vi "pco.camera_Avg_Example_IMAQ.vi"() -> ()   [LabVIEW 2019]
uses:
  pco.camera/Camera.lvclass
panel:
  out "rawImage":u16[][](array[numeric])
  out "Image":T1(plugin-control)
  in  "data_format":T2(ring)=enum."Mono16"
  out "Recorded Images":u32
  in  "Quit":bool
  in  "roiY1":u64=2 min=2 max=1040 step=1
  in  "roiX1":u64=2 min=2 max=1392 step=1
  in  "roiY0":u64=1 min=1 max=1039 step=1
  in  "roiX0":u64=1 min=1 max=1391 step=1
  out "Image Height":u64
  out "Image Width":u64
  in  "dwImgCount":u32=10 caption="Required Number of Images" max=4023
  out "Error":errorcluster {"code" format="%x"}
  # "This example shows how to continously compute and show an averaged image.\nHere the camera class is operated in sequence mode and the required number of images also defines the number of images that will be averaged\nIt is a good starting point for writing own applications.\nBut it will not be fail save, i.e. doesnt react on errors, just handles them forward to the end\n\nUsage:\nSelect your required image count you want to average over before you start the program.\nOnce started, the camera class will be initialized and image record will start automatically.\nInside the acquisition loop the program will record the image sequence.\nThen it calculates the average image and shows it.\nBy using the ROI parameters you can crop the image to select certain regions\n\nBy clicking Quit Application the record will stop and will force an exit of the camera class"
  # "pco.labview"
  # "Camera Setup"
  # "Recording Control"
  # "Parameters for image readout"
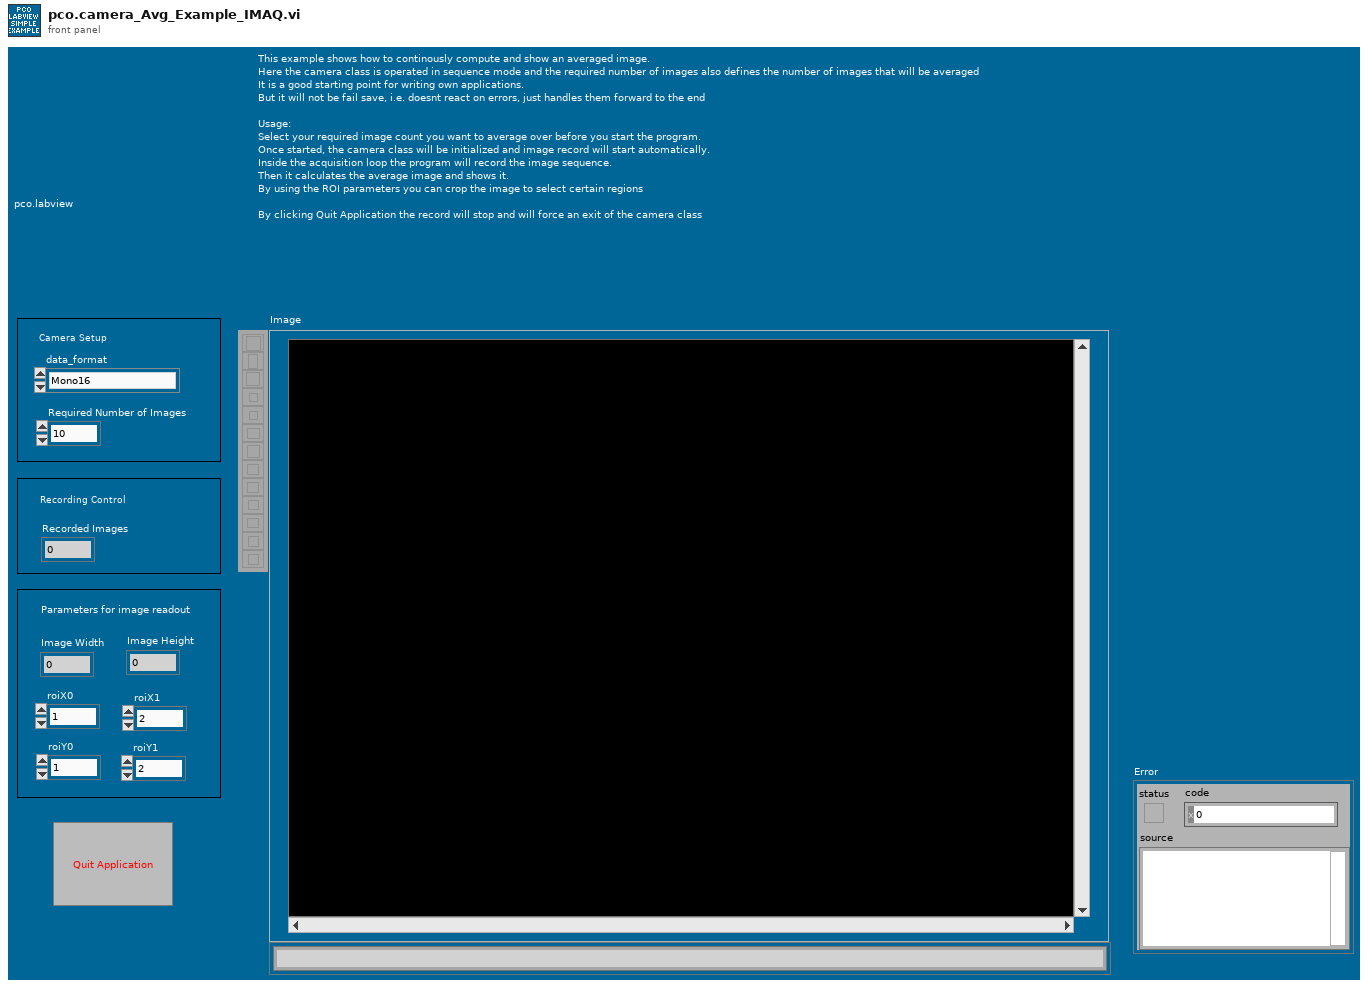
[diagram p1: front panel]
types:
  T1 = typedef "IMAQ Image.ctl" = refnum<image>
  T2 = enum16{"Undefined", "Mono8", "Mono16", "BGRA8", "RGBA8", "BGRA16", "RGBA16", "CompressedMono8"}
  T3 = enum8{"Enabled", "Disabled", "Disabled and Grayed Out"}
  T4 = enum16{"sequence", "sequence non blocking", "ring buffer", "fifo", "sequence_dpcore", "sequence_non_blocking_dpcore", "ring_buffer_dpcore", "fifo_dpcore", "tif", "multitif", "pcoraw", "b16", "dicom", "multidicom"}
  T5 = typedef "Image Type" = u32
  T6 = typedef "Camera.lvclass/binning.ctl" = cluster{"vert":u16, "horz":u16}
  T7 = cluster{"exposure_time_s":dbl, "delay_time_s":dbl, "roi":cluster{"x0":u64, "y0":u64, "x1":u64, "y1":u64}, "timestamp_mode":u16, "pixelrate":u32, "trigger_mode":u16, "acquire_mode":u16, "metadata_mode":u16, "noisefilter_mode":u16, "binning":T6}
  T8 = typedef "Color (U64)" = cluster{"Plane 3 (Blue)":u16, "Plane 2 (Green)":u16, "Plane 1 (Red)":u16, "Plane 4 (alpha)":u16}
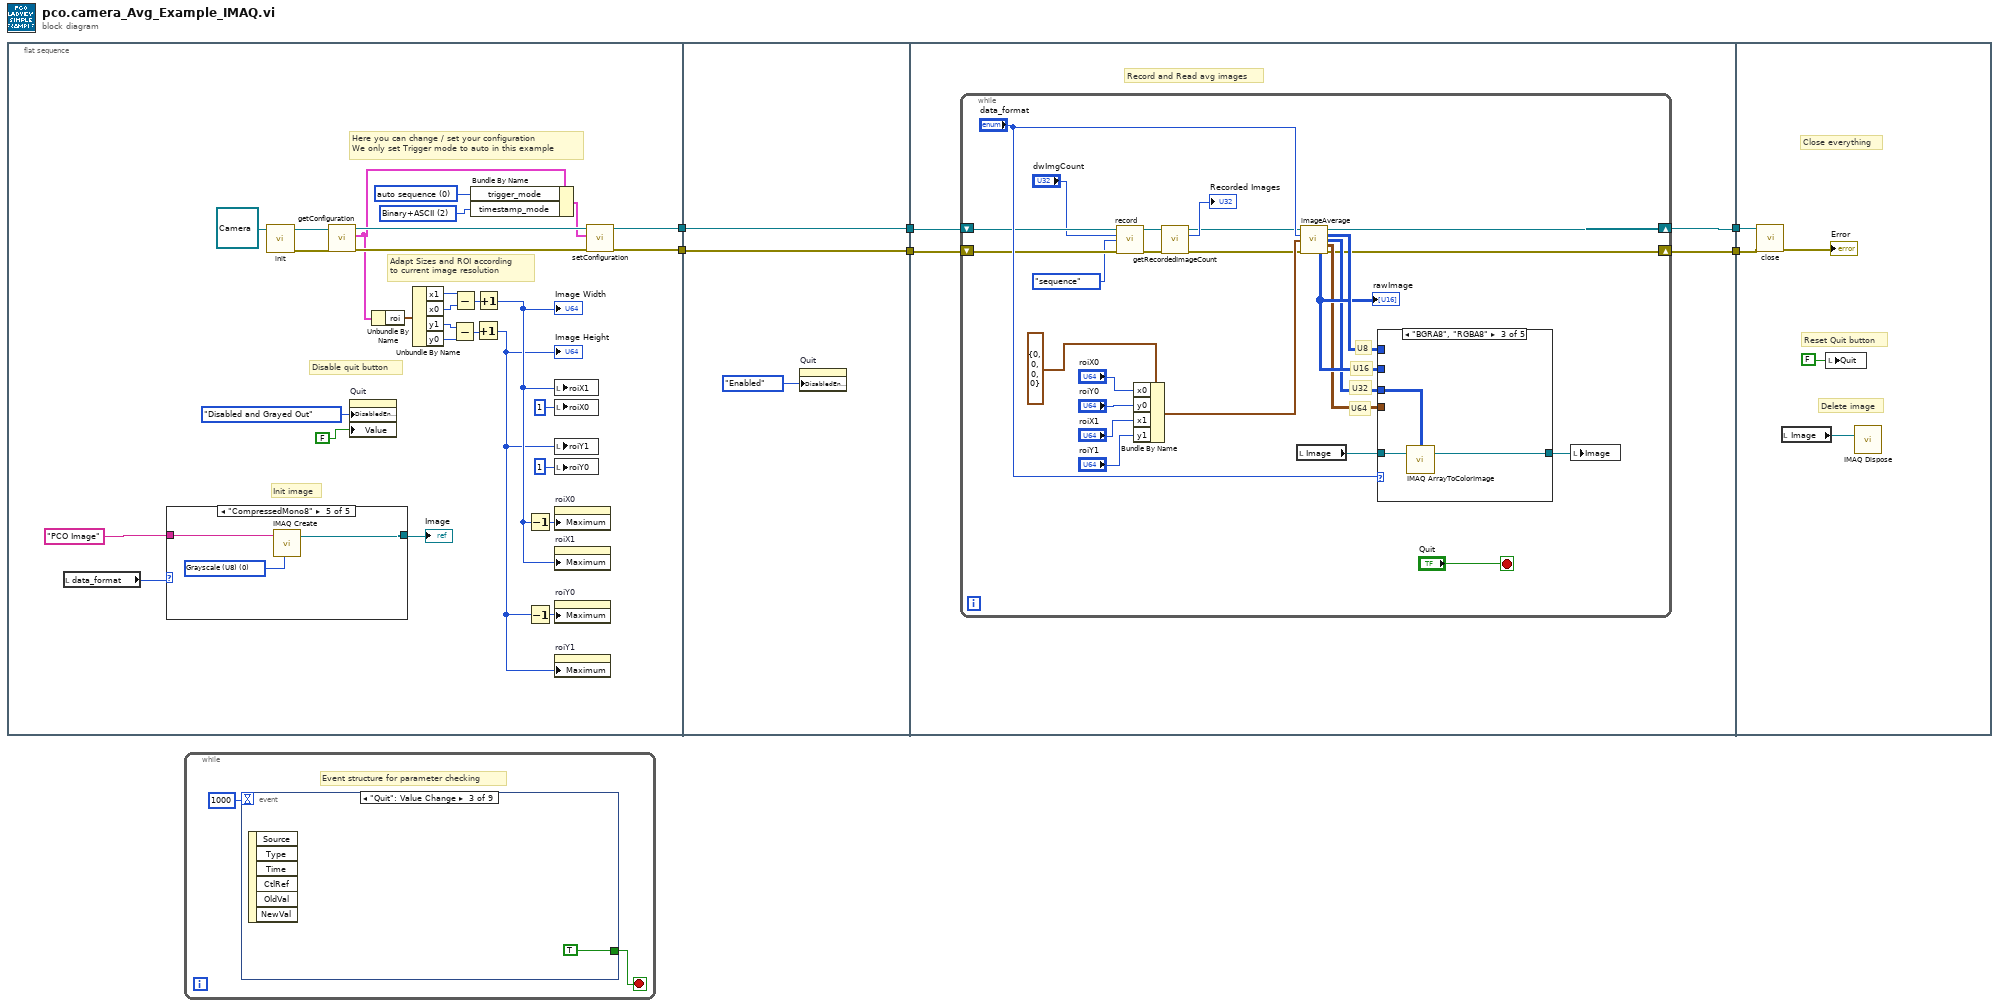
[diagram p0: block diagram]
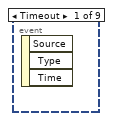
[diagram p2: hidden frame]
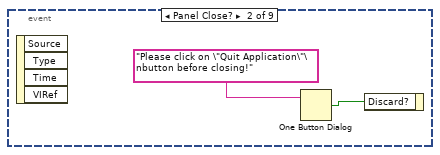
[diagram p3: hidden frame]
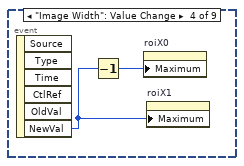
[diagram p4: hidden frame]
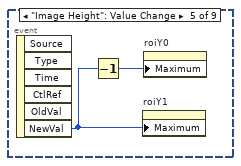
[diagram p5: hidden frame]
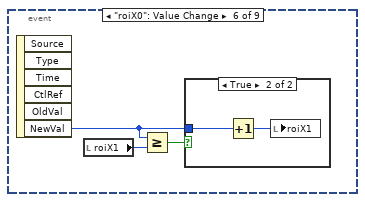
[diagram p6: hidden frame]
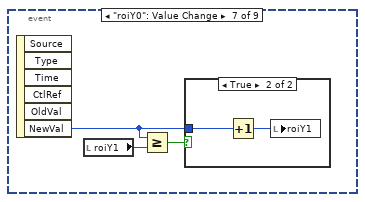
[diagram p8: hidden frame]
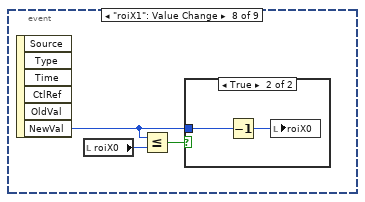
[diagram p10: hidden frame]
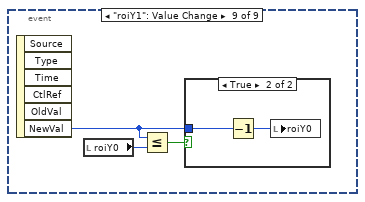
[diagram p12: hidden frame]
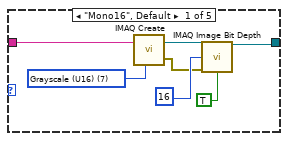
[diagram p14: hidden frame]
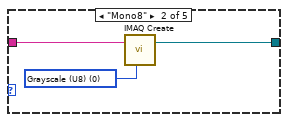
[diagram p15: hidden frame]
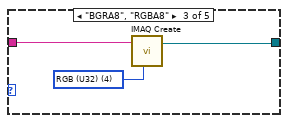
[diagram p16: hidden frame]
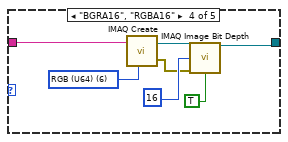
[diagram p17: hidden frame]
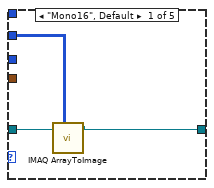
[diagram p18: hidden frame]
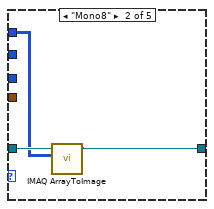
[diagram p19: hidden frame]
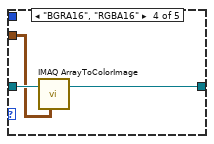
[diagram p20: hidden frame]
diagram:
  n1 = flat-sequence {
    tunnel: [w8] -> w6
    tunnel: [w7] -> w5
    tunnel: w6 -> [w60]
    tunnel: w5 -> [w59]
    tunnel: [w60] -> w4
    tunnel: [w59] -> w3
    tunnel: [w65] -> w2
    tunnel: [w64] -> w1
    tunnel: w3 -> [w63]
    tunnel: w4 -> [w62]
    tunnel: w2 -> [w108]
    tunnel: w1 -> [w107]
    frame #0 {
      w14 = u16 2 items=["OFF", "Binary", "Binary+ASCII", "ASCII"] ("TimestampMode")
      w32 = u16 0 items=["auto sequence"=0, "software trigger"=1, "external exposure start & software trigger"=2, "external exposure control"=3, "external synchronized"=4, "fast external exposure control"=5, "external CDS control"=6, "slow external exposure control"=7, "external synchronized HDSDI"=258] ("TriggerMode")
      # "Init image"
      # "Adapt Sizes and ROI according\nto current image resolution"
      # "Disable quit button"
      # "Here you can change / set your configuration\nWe only set Trigger mode to auto in this example"
      n2 = local read "data_format"() -> (w11:T2)
      n3 = case shown="\"CompressedMono8\"" w11 {
        tunnel: "PCO Image" ("Image Name") -> [w41 w45 w47 w54 w57]
        tunnel: [w36 w43 w46 w49 w56] -> w10
        frame "Mono16", Default {
          w42 = T5 7 items=["Grayscale (U8)", "Grayscale (I16)", "Grayscale (SGL)", "Complex (CSG)", "RGB (U32)", "HSL (U32)", "RGB (U64)", "Grayscale (U16)"] ("Image Type")
          n4 = call "IMAQ Create"("Image Name"=w41, "Image Type"=w42) -> ("New Image"=w38:T1, "error out"=w37:errorcluster)  [unwired: 3 in]
          n5 = call "IMAQ Image Bit Depth"("Image"=w38, "Bit Depth (0)"=u32 16, "error in (no error)"=w37, "Get/Set Bit Depth? (Set)"=TRUE) -> ("Image Out"=w36:T1)  [unwired: 9 in, 2 out]
        }
        frame "Mono8" {
          w44 = T5 0 items=["Grayscale (U8)", "Grayscale (I16)", "Grayscale (SGL)", "Complex (CSG)", "RGB (U32)", "HSL (U32)", "RGB (U64)", "Grayscale (U16)"] ("Image Type")
          n6 = call "IMAQ Create"("Image Name"=w45, "Image Type"=w44) -> ("New Image"=w43:T1)  [unwired: 3 in, 1 out]
        }
        frame "BGRA8", "RGBA8" {
          w48 = T5 4 items=["Grayscale (U8)", "Grayscale (I16)", "Grayscale (SGL)", "Complex (CSG)", "RGB (U32)", "HSL (U32)", "RGB (U64)", "Grayscale (U16)"] ("Image Type")
          n7 = call "IMAQ Create"("Image Name"=w47, "Image Type"=w48) -> ("New Image"=w46:T1)  [unwired: 3 in, 1 out]
        }
        frame "BGRA16", "RGBA16" {
          w55 = T5 6 items=["Grayscale (U8)", "Grayscale (I16)", "Grayscale (SGL)", "Complex (CSG)", "RGB (U32)", "HSL (U32)", "RGB (U64)", "Grayscale (U16)"] ("Image Type")
          n8 = call "IMAQ Create"("Image Name"=w54, "Image Type"=w55) -> ("New Image"=w51:T1, "error out"=w50:errorcluster)  [unwired: 3 in]
          n9 = call "IMAQ Image Bit Depth"("Image"=w51, "Bit Depth (0)"=u32 16, "error in (no error)"=w50, "Get/Set Bit Depth? (Set)"=TRUE) -> ("Image Out"=w49:T1)  [unwired: 9 in, 2 out]
        }
        frame "CompressedMono8" {
          w58 = T5 0 items=["Grayscale (U8)", "Grayscale (I16)", "Grayscale (SGL)", "Complex (CSG)", "RGB (U32)", "HSL (U32)", "RGB (U64)", "Grayscale (U16)"] ("Image Type")
          n10 = call "IMAQ Create"("Image Name"=w57, "Image Type"=w58) -> ("New Image"=w56:T1)  [unwired: 3 in, 1 out]
        }
      }
      "Image" <- w10
      n11 = call-dynamic "init.vi"("Camera in"=refnum<class "Camera.lvclass"> refnum ("PCOCamera in")) -> ("Camera out"=w34:refnum<class "Camera.lvclass">, "error out"=w33:errorcluster)  [unwired: 8 in]
      n12 = call-dynamic "getConfiguration.vi"("error in (no error)"=w33, "Camera in"=w34) -> ("error out"=w30:errorcluster, "configuration"=w24:T7, "Camera out"=w31:refnum<class "Camera.lvclass">)  [unwired: 7 in]
      n13 = property on="Quit" class="Bool (strict)"("DisabledEnum"=T3."Disabled and Grayed Out" ("Disabled"), "Value"=FALSE ("Stop")) -> ()  [unwired: 2 in, 2 out]
      n14 = Unbundle By Name(w24) -> ("roi"=w23:cluster{"x0":u64, "y0":u64, "x1":u64, "y1":u64})
      n15 = Unbundle By Name(w23) -> ("x1"=w21:u64, "x0"=w22:u64, "y1"=w19:u64, "y0"=w20:u64)
      n16 = Subtract(x=w19, y=w20) -> (x-y=w17:u64)
      n17 = Subtract(x=w21, y=w22) -> (x-y=w18:u64)
      n18 = Bundle By Name(cluster=w24, "trigger_mode"=w32, "timestamp_mode"=w14) -> (w29:T7)
      n19 = Increment(x=w17) -> (x+1=w15:u64)
      "Image Height" <- w15
      n20 = Increment(x=w18) -> (x+1=w16:u64)
      "Image Width" <- w16
      n21 = Decrement(x=w16) -> (x-1=w26:u64)
      n22 = Decrement(x=w15) -> (x-1=w25:u64)
      n23 = local write "roiX1"(w16) -> ()
      n24 = local write "roiX0"(u64 1 ("roiY0")) -> ()
      n25 = local write "roiY1"(w15) -> ()
      n26 = local write "roiY0"(u64 1 ("roiY0")) -> ()
      n27 = property on="roiX0" class="DigNum (strict)"("Maximum"=w26) -> ()  [unwired: 2 in, 2 out]
      n28 = property on="roiX1" class="DigNum (strict)"("Maximum"=w16) -> ()  [unwired: 2 in, 2 out]
      n29 = property on="roiY0" class="DigNum (strict)"("Maximum"=w25) -> ()  [unwired: 2 in, 2 out]
      n30 = property on="roiY1" class="DigNum (strict)"("Maximum"=w15) -> ()  [unwired: 2 in, 2 out]
      n31 = call-dynamic "setConfiguration.vi"("error in (no error)"=w30, "configuration"=w29, "Camera in"=w31) -> ("error out"=w7:errorcluster, "Camera out"=w8:refnum<class "Camera.lvclass">)  [unwired: 7 in]
    }
    frame #1 {
      n32 = property on="Quit" class="Bool (strict)"("DisabledEnum"=T3."Enabled" ("Disabled")) -> ()  [unwired: 2 in, 2 out]
    }
    frame #2 {
      # "Record and Read avg images"
      n33 = while {
        shift-right: [w76] -> w65
        shift-left: w62 -> [w75]
        shift-right: [w66] -> w64
        shift-left: w63 -> [w74]
        stop <- "Quit" stop-if-true
        # "U64"
        # "U32"
        # "U16"
        # "U8"
        n34 = call-dynamic "record.vi"("Camera in"=w75, "num_images"="dwImgCount", "record_mode"=T4."sequence", "error in (no error)"=w74) -> ("Camera out"=w72:refnum<class "Camera.lvclass">, "error out"=w71:errorcluster)  [unwired: 10 in]
        n35 = Bundle By Name(cluster=cluster{"x0":u64, "y0":u64, "x1":u64, "y1":u64} {"x0"=0, "y0"=0, "x1"=0, "y1"=0} ("roi"), "x0"="roiX0", "y0"="roiY0", "x1"="roiX1", "y1"="roiY1") -> (w86:cluster{"x0":u64, "y0":u64, "x1":u64, "y1":u64})
        n36 = call-dynamic "getRecordedImageCount.vi"("Camera in"=w72, "error in (no error)"=w71) -> ("Camera out"=w69:refnum<class "Camera.lvclass">, "recorded_image_count"=→"Recorded Images":u32, "error out"=w68:errorcluster)  [unwired: 11 in]
        n37 = local read "Image"() -> (w80:T1)
        n38 = call-dynamic "imageAverage.vi"("Camera in"=w69, "data_format"="data_format", "roi"=w86, "error in (no error)"=w68) -> ("Camera out"=w76:refnum<class "Camera.lvclass">, "image (U8)"=w84:u8[][], "image (U32)"=w82:u32[][], "image (U64)"=w81:T8[][], "raw_image (U16)"=w83:u16[][], "error out"=w66:errorcluster)  [unwired: 6 in]
        "rawImage" <- w83
        n39 = case shown="\"BGRA8\", \"RGBA8\"" "data_format" {
          tunnel: w80 -> [w93 w96 w99 w102 w105]
          tunnel: [w91 w94 w98 w100 w104] -> w79
          tunnel: w81 -> [_ _ _ w101 _]
          tunnel: w82 -> [_ _ w97 _ _]
          tunnel: w84 -> [_ w95 _ _ w103]
          tunnel: w83 -> [w92 _ _ _ _]
          frame "Mono16", Default {
            n40 = call "IMAQ ArrayToImage"("Image Pixels (U16)"=w92, "Image"=w93) -> ("Image Out"=w91:T1)  [unwired: 8 in, 1 out]
          }
          frame "Mono8" {
            n41 = call "IMAQ ArrayToImage"("Image Pixels (U8)"=w95, "Image"=w96) -> ("Image Out"=w94:T1)  [unwired: 8 in, 1 out]
          }
          frame "BGRA8", "RGBA8" {
            n42 = call "IMAQ ArrayToColorImage"("Image Pixels (U32)"=w97, "Image"=w99) -> ("Image Out"=w98:T1)  [unwired: 3 in, 1 out]
          }
          frame "BGRA16", "RGBA16" {
            n43 = call "IMAQ ArrayToColorImage"("Image"=w102, "Image Pixels (U64)"=w101) -> ("Image Out"=w100:T1)  [unwired: 3 in, 1 out]
          }
          frame "CompressedMono8" {
            n44 = call "IMAQ ArrayToImage"("Image Pixels (U8)"=w103, "Image"=w105) -> ("Image Out"=w104:T1)  [unwired: 8 in, 1 out]
          }
        }
        n45 = local write "Image"(w79) -> ()
      }
    }
    frame #3 {
      # "Delete image"
      # "Reset Quit button"
      # "Close everything"
      n46 = call-dynamic "close.vi"("error in (no error)"=w107, "Camera in"=w108) -> ("error out"=→"Error":errorcluster)  [unwired: 9 in]
      n47 = local read "Image"() -> (w106:T1)
      n48 = local write "Quit"(FALSE ("Stop")) -> ()
      n49 = call "IMAQ Dispose"("Image"=w106) -> ()  [unwired: 5 in, 1 out]
    }
  }
  n50 = while {
    stop <- w111 stop-if-true
    # "Event structure for parameter checking"
    n51 = event shown="[2] \"Quit\": Value Change" {
      selector: _ -> [_ _ _ _ _ _ _ _ _]
      dyn-events: _ -> [_ _ _ _ _ _ _ _ _]
      timeout: 1000 -> [_ _ _ _ _ _ _ _ _]
      tunnel: [_ _ TRUE _ _ _ _ _ _] -> w111
      event Timeout {
        n52 = event-data() -> ()  [unwired: 1 in, 3 out]
      }
      event Panel Close? {
        n53 = event-data() -> ()  [unwired: 1 in, 4 out]
        n54 = One Button Dialog(message="Please click on \"Quit Application\"\nbutton before closing!") -> (true=w113:bool)  [unwired: 1 in]
        n55 = event-data("Discard?"=w113) -> ()  [unwired: 1 in, 1 out]
      }
      event "Quit": Value Change {
        n56 = event-data() -> ()  [unwired: 1 in, 6 out]
      }
      event "Image Width": Value Change {
        n57 = event-data() -> ("NewVal"=w116:u64)  [unwired: 1 in, 5 out]
        n58 = Decrement(x=w116) -> (x-1=w117:u64)
        n59 = property on="roiX0" class="DigNum (strict)"("Maximum"=w117) -> ()  [unwired: 2 in, 2 out]
        n60 = property on="roiX1" class="DigNum (strict)"("Maximum"=w116) -> ()  [unwired: 2 in, 2 out]
      }
      event "Image Height": Value Change {
        n61 = event-data() -> ("NewVal"=w118:u64)  [unwired: 1 in, 5 out]
        n62 = Decrement(x=w118) -> (x-1=w119:u64)
        n63 = property on="roiY1" class="DigNum (strict)"("Maximum"=w118) -> ()  [unwired: 2 in, 2 out]
        n64 = property on="roiY0" class="DigNum (strict)"("Maximum"=w119) -> ()  [unwired: 2 in, 2 out]
      }
      event "roiX0": Value Change {
        n65 = event-data() -> ("NewVal"=w120:u64)  [unwired: 1 in, 5 out]
        n66 = local read "roiX1"() -> (w122:u64)
        n67 = Greater Or Equal?(x=w120, y=w122) -> (x >= y?=w121:bool)
        n68 = case shown="True" w121 {
          tunnel: w120 -> [_ w124]
          frame False {
          }
          frame True {
            n69 = Increment(x=w124) -> (x+1=w123:u64)
            n70 = local write "roiX1"(w123) -> ()
          }
        }
      }
      event "roiY0": Value Change {
        n71 = event-data() -> ("NewVal"=w125:u64)  [unwired: 1 in, 5 out]
        n72 = local read "roiY1"() -> (w127:u64)
        n73 = Greater Or Equal?(x=w125, y=w127) -> (x >= y?=w126:bool)
        n74 = case shown="True" w126 {
          tunnel: w125 -> [_ w129]
          frame False {
          }
          frame True {
            n75 = Increment(x=w129) -> (x+1=w128:u64)
            n76 = local write "roiY1"(w128) -> ()
          }
        }
      }
      event "roiX1": Value Change {
        n77 = event-data() -> ("NewVal"=w130:u64)  [unwired: 1 in, 5 out]
        n78 = local read "roiX0"() -> (w132:u64)
        n79 = Less Or Equal?(x=w130, y=w132) -> (x <= y?=w131:bool)
        n80 = case shown="True" w131 {
          tunnel: w130 -> [_ w134]
          frame False {
          }
          frame True {
            n81 = Decrement(x=w134) -> (x-1=w133:u64)
            n82 = local write "roiX0"(w133) -> ()
          }
        }
      }
      event "roiY1": Value Change {
        n83 = event-data() -> ("NewVal"=w135:u64)  [unwired: 1 in, 5 out]
        n84 = local read "roiY0"() -> (w137:u64)
        n85 = Less Or Equal?(x=w135, y=w137) -> (x <= y?=w136:bool)
        n86 = case shown="True" w136 {
          tunnel: w135 -> [_ w139]
          frame False {
          }
          frame True {
            n87 = Decrement(x=w139) -> (x-1=w138:u64)
            n88 = local write "roiY0"(w138) -> ()
          }
        }
      }
    }
  }
